vi "Calibration-Condition-RawCalData.vi"(11 "Raw Cal 1 Data In":dbl[](array[numeric])) -> (2 "sorted array of indexes":i32[](array[numeric]), 3 "conditioned Output Array":dbl[](array[numeric]))   [LabVIEW 2013, in "Calibration-RunTest.lvclass"]
uses:
  Calibration-RunTest.lvclass
panel:
  out "output array":dbl[](array[numeric])
  out "Value":dbl
  out "last good value":dbl
  out "Raw Input":dbl[](graph)
  out "conditioned Output":dbl[](graph)
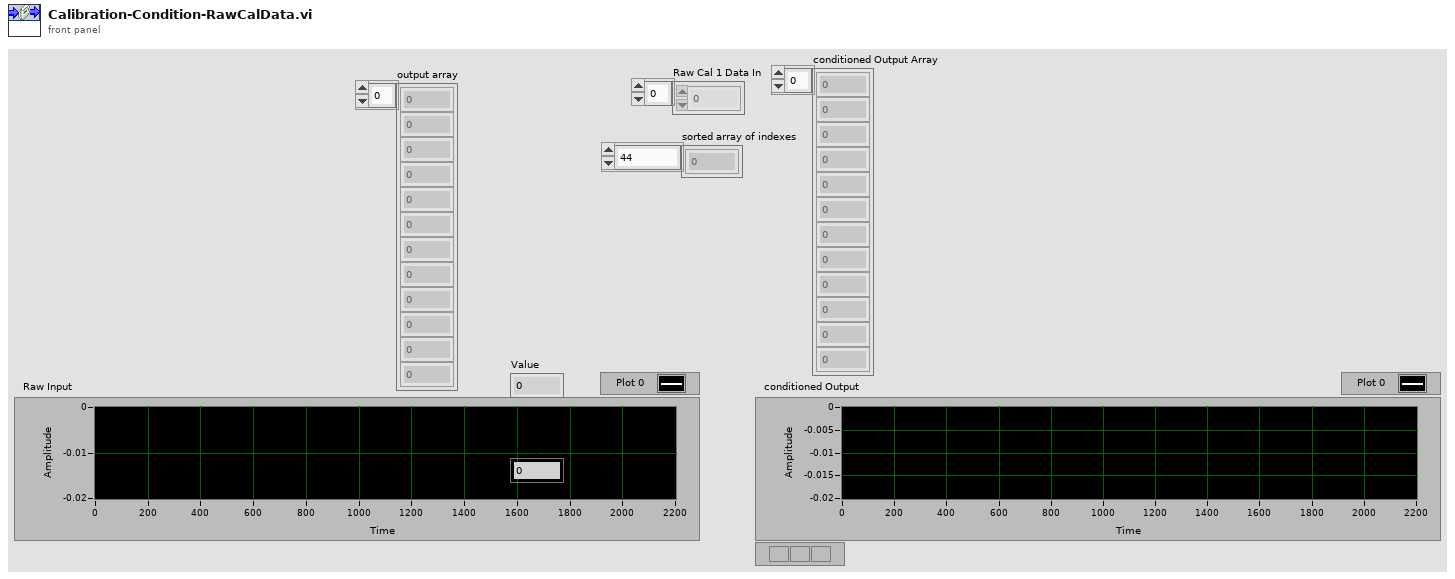
[diagram p1: front panel]
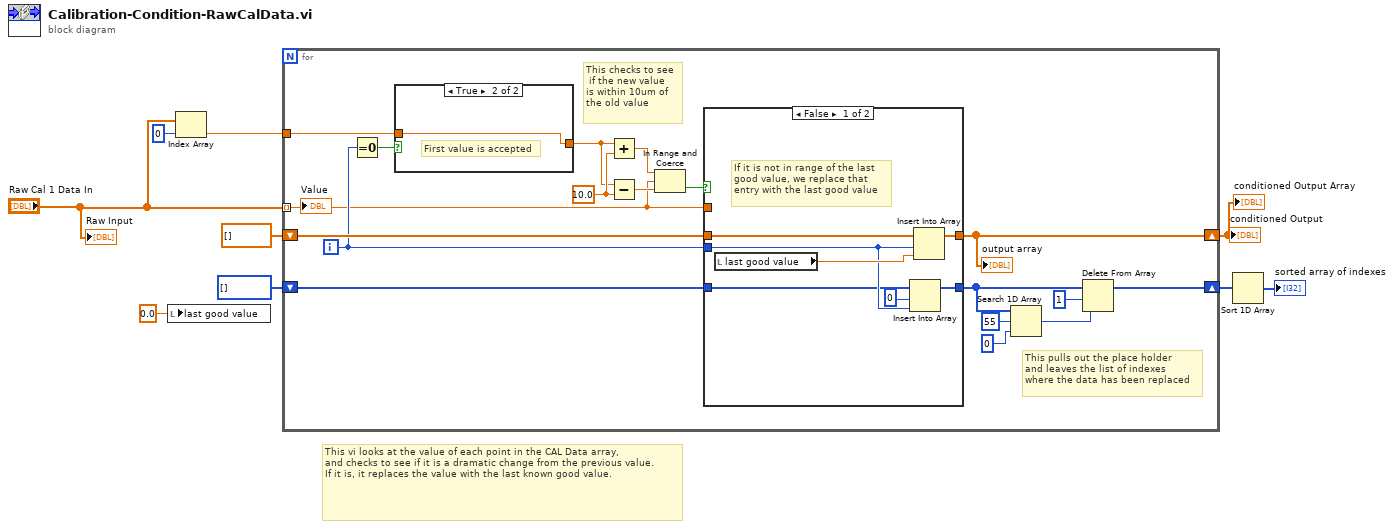
[diagram p0: block diagram]
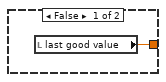
[diagram p2: hidden frame]
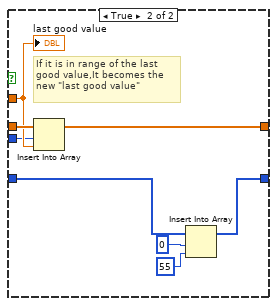
[diagram p3: hidden frame]
diagram:
  # "This vi looks at the value of each point in the CAL Data array,\nand checks to see if it is a dramatic change from the previous value.\nIf it is, it replaces the value with the last known good value."
  n1 = local write "last good value"(0.0 ("last good value")) -> ()
  n2 = Index Array(array="Raw Cal 1 Data In", index=0) -> (element=w6:dbl)
  n3 = for {
    tunnel: "Raw Cal 1 Data In" -> [w17] mode=indexing
    shift-right: [w27] -> w1
    shift-left: dbl[] [] -> [w26]
    tunnel: w6 -> [w20]
    shift-right: [w10] -> w9
    shift-left: i32[] [] -> [w16]
    i -> [w25]
    w19 = 10.0 ("Sensitivity")
    # "This pulls out the place holder\nand leaves the list of indexes\nwhere the data has been replaced"
    # "This checks to see\n if the new value\nis within 10um of \nthe old value"
    n4 = Equal To 0?(x=w25) -> (x = 0?=w24:bool)
    n5 = case shown="True" w24 {
      tunnel: [w28 w29] -> w18
      tunnel: w20 -> [_ w29]
      frame False {
        n6 = local read "last good value"() -> (w28:dbl)
      }
      frame True {
        # "First value is accepted"
      }
    }
    n7 = Add(x=w18, y=w19) -> (x+y=w22:dbl)
    n8 = Subtract(x=w18, y=w19) -> (x-y=w21:dbl)
    n9 = In Range and Coerce(upper limit=w22, x=w17, lower limit=w21) -> (In Range?=w23:bool)  [unwired: 1 out]
    n10 = case shown="False" w23 {
      tunnel: [w36 w44] -> w27
      tunnel: w26 -> [w35 w43]
      tunnel: w17 -> [_ w42]
      tunnel: w25 -> [w32 w41]
      tunnel: w16 -> [w31 w39]
      tunnel: [w30 w38] -> w11
      frame False {
        # "If it is not in range of the last \ngood value, we replace that \nentry with the last good value"
        n11 = local read "last good value"() -> (w34:dbl)
        n12 = Insert Into Array(array=w31, index=0, new element=w32) -> (w30:i32[])
        n13 = Insert Into Array(array=w35, index=w32, new element=w34) -> (w36:dbl[])
      }
      frame True {
        # "If it is in range of the last \ngood value,It becomes the \nnew \"last good value\""
        n14 = Insert Into Array(array=w43, index=w41, new element=w42) -> (w44:dbl[])
        n15 = Insert Into Array(array=w39, index=0, new element=55 ("new element/subarray")) -> (w38:i32[])
        "last good value" <- w42
      }
    }
    "output array" <- w27
    n16 = Search 1D Array(1D array=w11, element=55, start index (0)=0) -> (index of element=w15:i32)
    n17 = Delete From Array(array=w11, length=1, index=w15) -> (array with subset deleted=w10:i32[])  [unwired: 1 out]
    "Value" <- w17
  }
  "conditioned Output" <- w1
  "conditioned Output Array" <- w1
  n18 = Sort 1D Array(array=w9) -> (sorted array=→"sorted array of indexes":i32[])
  "Raw Input" <- "Raw Cal 1 Data In"
